vi "load target with engines.vi"(8 "error in (no error)":errorcluster, 9 "target alias":string, 10 "engine aliases (empty = ALL)":string[](array[string]), 11 "file path":path) -> (0 "error out":errorcluster, 2 "engines":T1[](array[typedef]), 3 "PL_Target Configuration out":refnum<class "PL_Target Configuration.lvclass">)   [LabVIEW 2014, in "PL_Target Runtime.lvclass"]
uses:
  PL_Target Runtime.lvclass
  platypus configuration/engines cluster.ctl
  <vilib>/NI/Module Execution Interface/Engine Configuration/engine configuration.lvclass
  <vilib>/NI/Tag Bus Module Framework/module configuration/TBM module configuration.lvclass
  target configuration/PL_Target Configuration.lvclass
  <vilib>/NI/Configuration Framework/tree serializer/NISE_CEF_TreeSerializer.lvlib
  flattened data interface/PL_Serialization Interface.lvlib
  <vilib>/NI/Configuration Framework/serializable configuration/NISE_CEF_serializable configuration.lvclass
  platypus configuration/PLConfigurationSerializer.lvlib
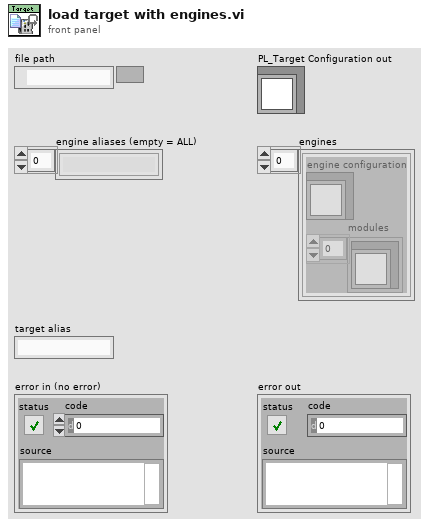
[diagram p1: front panel]
types:
  T1 = typedef "PLConfigurationSerializer.lvlib/engines cluster.ctl" = cluster{"engine configuration":refnum<class "engine configuration.lvclass">, "modules":refnum<class "TBM module configuration.lvclass">[]}
  T2 = typedef "NISE_CEF_TreeSerializer.lvlib/base file format.ctl" = cluster{"version":string, "data":string}
  T3 = typedef "NISE_CEF_TreeSerializer.lvlib/flat hierarchy.ctl" = cluster{"hierarchy structure":T4, "instance data":T6[]}
  T4 = typedef "NISE_CEF_TreeSerializer.lvlib/full hierarchy.ctl" = cluster{"root":string, "hierarchy":T5[]}
  T5 = typedef "NISE_CEF_TreeSerializer.lvlib/hierarchy element.ctl" = cluster{"current node":string, "children":string[]}
  T6 = typedef "NISE_CEF_TreeSerializer.lvlib/instance data.ctl" = cluster{"ID":string, "Alias":string, "class":string, "version":string, "data":string}
  T7 = typedef "PLConfigurationSerializer.lvlib/targets cluster.ctl" = cluster{"Target Configuration":refnum<class "PL_Target Configuration.lvclass">, "engines":T1[]}
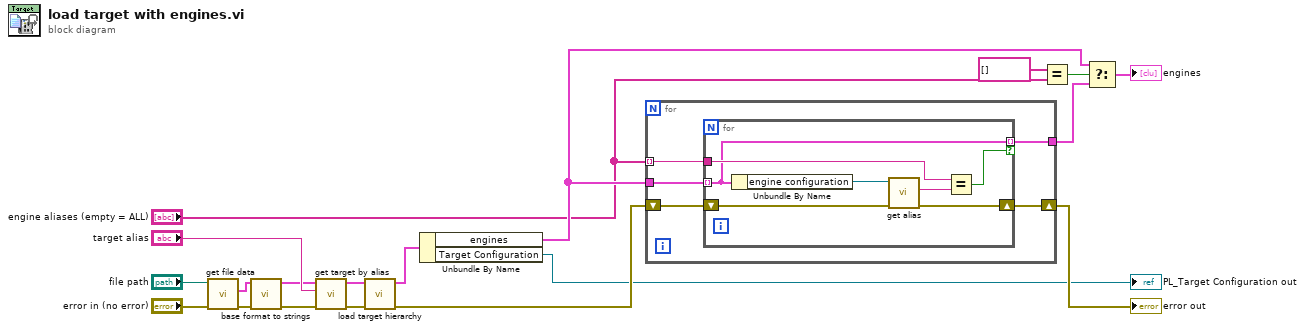
[diagram p0: block diagram]
diagram:
  n1 = call <vilib>:"get file data.vi"("error in"="error in (no error)", "Path"="file path") -> ("error out"=w2:errorcluster, "format"=w1:T2)  [unwired: 8 in]
  n2 = call <vilib>:"base format to strings.vi"("error in"=w2, "format"=w1) -> ("error out"=w5:errorcluster, "data"=w4:T3)  [unwired: 8 in]
  n3 = call "get target by alias.vi"("error in"=w5, "alias"="target alias", "system hierarchy"=w4) -> ("error out"=w8:errorcluster, "target hierarchy"=w7:T3)  [unwired: 7 in]
  n4 = call "load target hierarchy.vi"("error in"=w8, "target hierarchy"=w7) -> ("error out"=w19:errorcluster, "targets cluster out"=w9:T7)  [unwired: 8 in]
  n5 = Unbundle By Name(w9) -> ("engines"=w14:T1[], "Target Configuration"=→"PL_Target Configuration out":refnum<class "PL_Target Configuration.lvclass">)
  n6 = for {
    tunnel: w14 -> [w24]
    tunnel: "engine aliases (empty = ALL)" -> [w21] mode=indexing
    shift-right: [w22] -> w18
    shift-left: w19 -> [w23]
    tunnel: [w20] -> w15
    n7 = for {
      tunnel: w24 -> [w26] mode=indexing
      shift-right: [w29] -> w22
      shift-left: w23 -> [w30]
      tunnel: w21 -> [w27]
      tunnel: [w26] -> w20 mode=indexing if=w25
      n8 = Unbundle By Name(w26) -> ("engine configuration"=w31:refnum<class "engine configuration.lvclass">)
      n9 = call <vilib>:"get alias.vi"("error in"=w30, "configuration in"=w31) -> ("error out"=w29:errorcluster, "alias"=w28:string)  [unwired: 7 in, 1 out]
      n10 = Equal?(x=w27, y=w28) -> (x = y?=w25:bool)
    }
  }
  "error out" <- w18
  n11 = Equal?(x=string[] [], y="engine aliases (empty = ALL)") -> (x = y?=w13:bool)
  n12 = Select(t=w14, s=w13, f=w15) -> (s? t:f=→"engines":T1[])
